vi "Init Control.vi"(5 "Group":refnum<class "Group DBL.lvclass">, 6 "Period ms":i64, 7 "VolatusAPI":refnum<class "VolatusAPI.lvclass">, 8 "error in (no error)":errorcluster, 9 "Control MsgQ":refnum<class "MessageQ.lvclass">, 10 "Config Element":refnum<class "Config Element.lvclass">, 11 "SequencedValves in":refnum<class "TriggerDelayControl.lvclass">) -> (0 "error out":errorcluster, 3 "SequencedValves out":refnum<class "TriggerDelayControl.lvclass">)   [LabVIEW 2020, in "VolatusControl.lvlib" / "TriggerDelayControl.lvclass"]
uses:
  TriggerDelayControl.lvclass
  lv-cdm/CDM-Config/Config Element/Config Element.lvclass
  Volatus/VolatusAPI/VolatusAPI.lvclass
  Volatus/MessageQ/MessageQ.lvclass
  lv-vecto/Vecto/Group DBL/Group DBL.lvclass
  C:/dev/lv20CE/relink/lv-vecto/Vecto/Group/Group.lvclass
  TriggerDelayControl.lvclass/TriggerDelayControl.ctl
  lv-cdm/CDM-Config/Config Element/Owner.vi
  lv-cdm/CDM-Config/Config Manager/Lookup Descendant.vi
  lv-cdm/CDM-Config/Config Filter/Config Lookup.lvclass
  lv-vecto/Vecto/Group/Group.lvclass
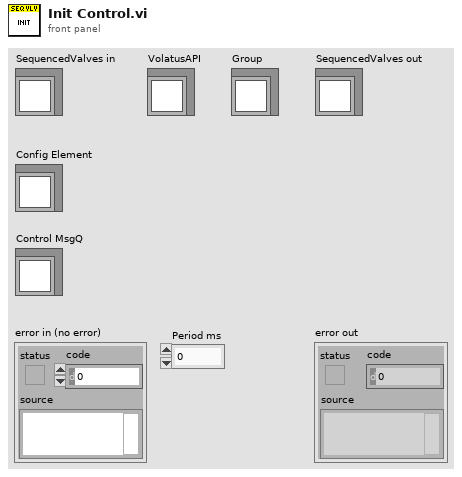
[diagram p1: front panel]
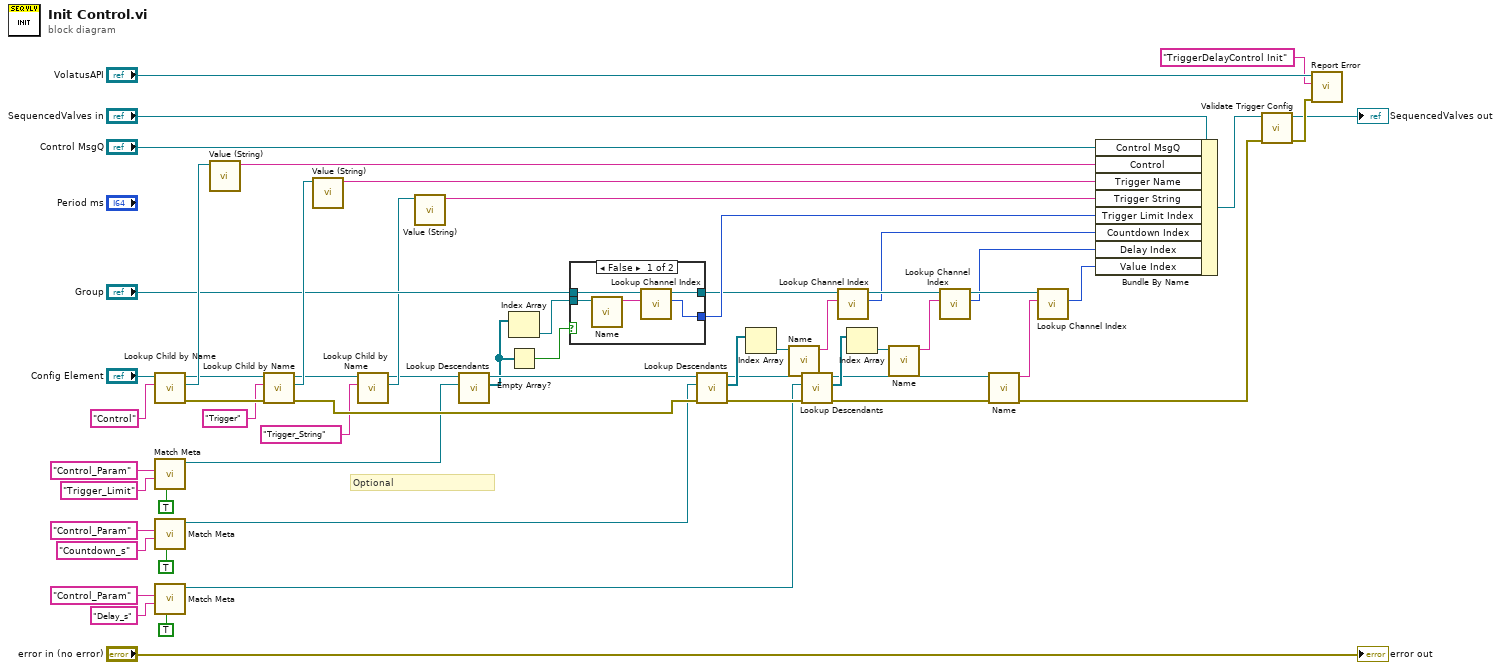
[diagram p0: block diagram]
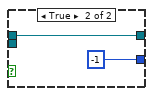
[diagram p2: hidden frame]
diagram:
  # "Optional"
  n1 = call "Lookup Child by Name.vi"("Name"="Control", "Config Element in"="Config Element") -> ("error out"=w26:errorcluster, "Child"=w54:refnum<class "Config Element.lvclass">, "Config Element out"=w27:refnum<class "Config Element.lvclass">)  [unwired: 6 in, 1 out]
  n2 = call "Match Meta.vi"("Exact Value (F)"=TRUE, "Value (Any)"="Trigger_Limit" ("Name"), "Name"="Control_Param") -> ("Config Lookup out"=w19:refnum<class "Config Lookup.lvclass">)  [unwired: 7 in, 1 out]
  n3 = call "Match Meta.vi"("Exact Value (F)"=TRUE, "Value (Any)"="Countdown_s" ("Name"), "Name"="Control_Param") -> ("Config Lookup out"=w33:refnum<class "Config Lookup.lvclass">)  [unwired: 7 in, 1 out]
  n4 = call "Match Meta.vi"("Exact Value (F)"=TRUE, "Value (Any)"="Delay_s" ("Name"), "Name"="Control_Param") -> ("Config Lookup out"=w51:refnum<class "Config Lookup.lvclass">)  [unwired: 7 in, 1 out]
  n5 = call "Value (String).vi"("Config Element in"=w54) -> ("String Value"=w49:string)  [unwired: 9 in, 1 out]
  n6 = call "Lookup Child by Name.vi"("error in (no error)"=w26, "Name"="Trigger", "Config Element in"=w27) -> ("error out"=w57:errorcluster, "Child"=w24:refnum<class "Config Element.lvclass">, "Config Element out"=w11:refnum<class "Config Element.lvclass">)  [unwired: 5 in, 1 out]
  n7 = call "Value (String).vi"("Config Element in"=w24) -> ("String Value"=w23:string)  [unwired: 9 in, 1 out]
  n8 = call "Lookup Child by Name.vi"("Name"="Trigger_String", "Config Element in"=w11) -> ("Child"=w10:refnum<class "Config Element.lvclass">, "Config Element out"=w8:refnum<class "Config Element.lvclass">)  [unwired: 6 in, 2 out]
  n9 = call "Value (String).vi"("Config Element in"=w10) -> ("String Value"=w9:string)  [unwired: 9 in, 1 out]
  n10 = call "Lookup Descendants.vi"("Lookup"=w19, "Config Element in"=w8) -> ("Descendants"=w7:refnum<class "Config Element.lvclass">[], "Config Element out"=w17:refnum<class "Config Element.lvclass">)  [unwired: 7 in, 1 out]
  n11 = Index Array(array=w7) -> (element=w18:refnum<class "Config Element.lvclass">)  [unwired: 1 in]
  n12 = Empty Array?(array=w7) -> (empty?=w6:bool)
  n13 = case shown="False" w6 {
    tunnel: w18 -> [w62 _]
    tunnel: [w61 -1 ("Index")] -> w15
    tunnel: "Group" -> [w60 w65]
    tunnel: [w59 w65] -> w13
    frame False {
      n14 = call "Name.vi"("Config Element in"=w62) -> ("Name"=w63:string)  [unwired: 9 in, 1 out]
      n15 = call "Lookup Channel Index.vi"("Channel Name"=w63, "GroupAbstract in"=w60) -> ("Index"=w61:i32, "GroupAbstract out"=w59:refnum<class "Group DBL.lvclass">)  [unwired: 7 in, 1 out]
    }
    frame True {
    }
  }
  n16 = call "Lookup Descendants.vi"("error in (no error)"=w57, "Lookup"=w33, "Config Element in"=w17) -> ("error out"=w56:errorcluster, "Descendants"=w32:refnum<class "Config Element.lvclass">[], "Config Element out"=w16:refnum<class "Config Element.lvclass">)  [unwired: 6 in]
  n17 = Index Array(array=w32) -> (element=w30:refnum<class "Config Element.lvclass">)  [unwired: 1 in]
  n18 = call "Name.vi"("Config Element in"=w30) -> ("Name"=w29:string)  [unwired: 9 in, 1 out]
  n19 = call "Lookup Descendants.vi"("error in (no error)"=w56, "Lookup"=w51, "Config Element in"=w16) -> ("error out"=w3:errorcluster, "Descendants"=w50:refnum<class "Config Element.lvclass">[], "Config Element out"=w47:refnum<class "Config Element.lvclass">)  [unwired: 6 in]
  n20 = call "Lookup Channel Index.vi"("Channel Name"=w29, "GroupAbstract in"=w13) -> ("Index"=w28:i32, "GroupAbstract out"=w31:refnum<class "Group DBL.lvclass">)  [unwired: 7 in, 1 out]
  n21 = Index Array(array=w50) -> (element=w46:refnum<class "Config Element.lvclass">)  [unwired: 1 in]
  n22 = call "Name.vi"("Config Element in"=w46) -> ("Name"=w45:string)  [unwired: 9 in, 1 out]
  n23 = call "Lookup Channel Index.vi"("Channel Name"=w45, "GroupAbstract in"=w31) -> ("Index"=w38:i32, "GroupAbstract out"=w44:refnum<class "Group DBL.lvclass">)  [unwired: 7 in, 1 out]
  n24 = call "Name.vi"("Config Element in"=w47) -> ("Name"=w43:string)  [unwired: 9 in, 1 out]
  n25 = call "Lookup Channel Index.vi"("Channel Name"=w43, "GroupAbstract in"=w44) -> ("Index"=w37:i32)  [unwired: 7 in, 2 out]
  n26 = Bundle By Name(cluster="SequencedValves in", "Control MsgQ"="Control MsgQ", "Control"=w49, "Trigger Name"=w23, "Trigger String"=w9, "Trigger Limit Index"=w15, "Countdown Index"=w28, "Delay Index"=w38, "Value Index"=w37) -> (w41:refnum<class "TriggerDelayControl.lvclass">)
  n27 = call "Validate Trigger Config.vi"("error in (no error)"=w3, "TriggerDelayControl in"=w41) -> ("error out"=w58:errorcluster, "TriggerDelayControl out"=→"SequencedValves out":refnum<class "TriggerDelayControl.lvclass">)  [unwired: 8 in]
  n28 = call "Report Error.vi"("error in (no error)"=w58, "Context"="TriggerDelayControl Init", "VolatusAPI in"="VolatusAPI") -> ()  [unwired: 7 in, 2 out]
  "error out" <- "error in (no error)"
